vi "RTS Extract Point Array.vi"(8 "Error In":errorcluster, 10 "Chamber Data in":string[][](array[string])=[["System Date", "System Time", "Elapsed Time (sec)", "Elapsed Time (hrs)", "Voltage (V)", "RMS Current (Amps)", "Power (Watts)", "Watt Hours (Wh)", "Voltage Total Harmonic Distortion (%)", "Frequency (Hz)", "Apparent Power (VA)", "Power Factor", "TC 1", "TC 2", "TC 3", "TC 4", "TC 5", "TC 6", "TC 7", "TC 8", "TC 9", "TC 10", "TC 11", "TC 12", "TC 13", "TC 14", "TC 15", "TC 16", "TC 17", "TC 18", "TC 19", "TC 20", "TC 21", "TC 22", "TC 23", "TC 24", "TC 25", "TC 26", "TC 27", "TC 28", "TC 29", "TC 30", "AUX 1", "AUX 2", "CAL CL", "Room Setpoint Temperature", "Room Setpoint Humidity", "Room Temperature (°F)", "Room Humidity (%)", "Door Enable", "Room Setpoint Cool Temperature", "Room Setpoint Dehumidification Temperature", "Supply Temperature (°F)", "Cool Temperature (°F)", "Dehumidification Temperature (°F)", "Glycol Temperature (°F)", "Heat Rate (%)", "Steam Rate (%)", "Cool Rate (%)", "Dehumidification Rate (%)", "Room Status", "Room Dry P", "Room Dry I", "Room Humidity P", "Room Humidity I", "Room Heat P", "Room Heat I", "Room Cool Temperature P", "Room Cool Temperature I", "Room Dehumidification Temperature P", "Room Dehumidification Temperature I", "Voltage Setpoint 1", "60 Hz Power", "50 Hz Power", "120V Range", "240V Range", "Ground Line", "Ground Neutral", "Measure Ground Leakage Current", "Room OK", "S1 Freezer Relay", "S1 Cab Relay", "S1 Slide Relay", "Recording Data", "CVS Location", "Point Location"], ["01/24/2018", "06:36:24.375", "0.000000", "0.000000", "115.046623", "0.030182", "0.135573", "964.507616", "3.000000", "60.021709", "3.472371", "1.000000", "-2.310000", "-1.920000", "-0.910000", "327.670000", "327.670000", "327.670000", "327.670000", "327.670000", "327.670000", "327.670000", "38.020000", "35.660000", "35.030000", "327.670000", "327.670000", "327.670000", "327.670000", "327.670000", "327.670000", "327.670000", "327.670000", "327.670000", "327.670000", "70.360000", "327.670000", "327.670000", "70.300000", "327.670000", "32767.000000", "32767.000000", "0.001000", "0.000000", "1.988000", "70.000000", "35.000000", "70.040000", "38.150000", "1.000000", "55.000000", "48.000000", "66.700000", "55.180000", "48.160000", "0.000000", "36.920000", "0.000000", "30.630000", "8.240000", "0.000000", "200.000000", "15000.000000", "400.000000", "15000.000000", "1000.000000", "2000.000000", "500.000000", "6000.000000", "500.000000", "6000.000000", "115.000000", "1.000000", "0.000000", "1.000000", "0.000000", "0.000000", "1.000000", "0.000000", "1.000000", "0.000000", "0.000000", "0.000000", "FALSE", "", ""], ["System Date", "System Time", "Elapsed Time (sec)", "Elapsed Time (hrs)", "Voltage (V)", "RMS Current (Amps)", "Power (Watts)", "Watt Hours (Wh)", "Voltage Total Harmonic Distortion (%)", "Frequency (Hz)", "Apparent Power (VA)", "Power Factor", "TC 1", "TC 2", "TC 3", "TC 4", "TC 5", "TC 6", "TC 7", "TC 8", "TC 9", "TC 10", "TC 11", "TC 12", "TC 13", "TC 14", "TC 15", "TC 16", "TC 17", "TC 18", "TC 19", "TC 20", "TC 21", "TC 22", "TC 23", "TC 24", "TC 25", "TC 26", "TC 27", "TC 28", "TC 29", "TC 30", "AUX 1", "AUX 2", "CAL CL", "Room Setpoint Temperature", "Room Setpoint Humidity", "Room Temperature (°F)", "Room Humidity (%)", "Door Enable", "Room Setpoint Cool Temperature", "Room Setpoint Dehumidification Temperature", "Supply Temperature (°F)", "Cool Temperature (°F)", "Dehumidification Temperature (°F)", "Glycol Temperature (°F)", "Heat Rate (%)", "Steam Rate (%)", "Cool Rate (%)", "Dehumidification Rate (%)", "Room Status", "Room Dry P", "Room Dry I", "Room Humidity P", "Room Humidity I", "Room Heat P", "Room Heat I", "Room Cool Temperature P", "Room Cool Temperature I", "Room Dehumidification Temperature P", "Room Dehumidification Temperature I", "Voltage Setpoint 2", "60 Hz Power", "50 Hz Power", "120V Range", "240V Range", "Ground Line", "Ground Neutral", "Measure Ground Leakage Current", "Fault", "S2 Freezer Relay", "S2 Cab Relay", "S2 Slide Relay", "Recording Data", "CVS Location", "Point Location"], ["01/24/2018", "06:36:24.375", "0.000000", "0.000000", "114.863785", "0.030740", "0.139474", "26203.680290", "3.500000", "60.021633", "3.530865", "1.000000", "10.000000", "8.600000", "8.210000", "327.670000", "327.670000", "327.670000", "327.670000", "327.670000", "327.670000", "327.670000", "41.900000", "42.090000", "43.130000", "327.670000", "327.670000", "327.670000", "327.670000", "327.670000", "327.670000", "327.670000", "327.670000", "327.670000", "327.670000", "69.920000", "327.670000", "327.670000", "70.410000", "327.670000", "32767.000000", "32767.000000", "0.001000", "0.001000", "1.991000", "70.000000", "35.000000", "70.040000", "38.150000", "1.000000", "55.000000", "48.000000", "66.700000", "55.180000", "48.160000", "0.000000", "36.920000", "0.000000", "30.630000", "8.240000", "0.000000", "200.000000", "15000.000000", "400.000000", "15000.000000", "1000.000000", "2000.000000", "500.000000", "6000.000000", "500.000000", "6000.000000", "115.000000", "1.000000", "0.000000", "1.000000", "0.000000", "0.000000", "1.000000", "0.000000", "0.000000", "0.000000", "0.000000", "0.000000", "FALSE", "", ""], ["System Date", "System Time", "Elapsed Time (sec)", "Elapsed Time (hrs)", "Voltage (V)", "RMS Current (Amps)", "Power (Watts)", "Watt Hours (Wh)", "Voltage Total Harmonic Distortion (%)", "Frequency (Hz)", "Apparent Power (VA)", "Power Factor", "TC 1", "TC 2", "TC 3", "TC 4", "TC 5", "TC 6", "TC 7", "TC 8", "TC 9", "TC 10", "TC 11", "TC 12", "TC 13", "TC 14", "TC 15", "TC 16", "TC 17", "TC 18", "TC 19", "TC 20", "TC 21", "TC 22", "TC 23", "TC 24", "TC 25", "TC 26", "TC 27", "TC 28", "TC 29", "TC 30", "AUX 1", "AUX 2", "CAL CL", "Room Setpoint Temperature", "Room Setpoint Humidity", "Room Temperature (°F)", "Room Humidity (%)", "Door Enable", "Room Setpoint Cool Temperature", "Room Setpoint Dehumidification Temperature", "Supply Temperature (°F)", "Cool Temperature (°F)", "Dehumidification Temperature (°F)", "Glycol Temperature (°F)", "Heat Rate (%)", "Steam Rate (%)", "Cool Rate (%)", "Dehumidification Rate (%)", "Room Status", "Room Dry P", "Room Dry I", "Room Humidity P", "Room Humidity I", "Room Heat P", "Room Heat I", "Room Cool Temperature P", "Room Cool Temperature I", "Room Dehumidification Temperature P", "Room Dehumidification Temperature I", "Voltage Setpoint 3", "60 Hz Power", "50 Hz Power", "120V Range", "240V Range", "Ground Line", "Ground Neutral", "Measure Ground Leakage Current", "Room Heat", "S3 Freezer Relay", "S3 Cab Relay", "S3 Slide Relay", "Recording Data", "CVS Location", "Point Location"], ["01/24/2018", "06:36:24.376", "0.000000", "0.000000", "114.844543", "0.030078", "0.135316", "27955.201782", "3.100000", "60.022556", "3.456682", "1.000000", "0.690000", "0.850000", "2.060000", "327.670000", "327.670000", "327.670000", "327.670000", "327.670000", "327.670000", "327.670000", "37.750000", "38.160000", "38.080000", "327.670000", "327.670000", "327.670000", "327.670000", "327.670000", "327.670000", "327.670000", "327.670000", "327.670000", "327.670000", "70.410000", "327.670000", "327.670000", "70.770000", "327.670000", "32767.000000", "32767.000000", "0.001000", "0.001000", "1.963000", "70.000000", "35.000000", "70.040000", "38.150000", "1.000000", "55.000000", "48.000000", "66.700000", "55.180000", "48.160000", "0.000000", "36.920000", "0.000000", "30.630000", "8.240000", "0.000000", "200.000000", "15000.000000", "400.000000", "15000.000000", "1000.000000", "2000.000000", "500.000000", "6000.000000", "500.000000", "6000.000000", "115.000000", "1.000000", "0.000000", "1.000000", "0.000000", "0.000000", "1.000000", "0.000000", "1.000000", "0.000000", "0.000000", "0.000000", "FALSE", "", ""], ["System Date", "System Time", "Elapsed Time (sec)", "Elapsed Time (hrs)", "Voltage (V)", "RMS Current (Amps)", "Power (Watts)", "Watt Hours (Wh)", "Voltage Total Harmonic Distortion (%)", "Frequency (Hz)", "Apparent Power (VA)", "Power Factor", "TC 1", "TC 2", "TC 3", "TC 4", "TC 5", "TC 6", "TC 7", "TC 8", "TC 9", "TC 10", "TC 11", "TC 12", "TC 13", "TC 14", "TC 15", "TC 16", "TC 17", "TC 18", "TC 19", "TC 20", "TC 21", "TC 22", "TC 23", "TC 24", "TC 25", "TC 26", "TC 27", "TC 28", "TC 29", "TC 30", "AUX 1", "AUX 2", "CAL CL", "Room Setpoint Temperature", "Room Setpoint Humidity", "Room Temperature (°F)", "Room Humidity (%)", "Door Enable", "Room Setpoint Cool Temperature", "Room Setpoint Dehumidification Temperature", "Supply Temperature (°F)", "Cool Temperature (°F)", "Dehumidification Temperature (°F)", "Glycol Temperature (°F)", "Heat Rate (%)", "Steam Rate (%)", "Cool Rate (%)", "Dehumidification Rate (%)", "Room Status", "Room Dry P", "Room Dry I", "Room Humidity P", "Room Humidity I", "Room Heat P", "Room Heat I", "Room Cool Temperature P", "Room Cool Temperature I", "Room Dehumidification Temperature P", "Room Dehumidification Temperature I", "Voltage Setpoint 4", "60 Hz Power", "50 Hz Power", "120V Range", "240V Range", "Ground Line", "Ground Neutral", "Measure Ground Leakage Current", "Room Blower", "S4 Freezer Relay", "S4 Cab Relay", "S4 Slide Relay", "Recording Data", "CVS Location", "Point Location"], ["01/24/2018", "06:36:24.376", "0.000000", "0.000000", "115.200577", "0.030417", "0.136655", "26339.492026", "3.200000", "60.021862", "3.504017", "1.000000", "1.700000", "3.490000", "4.180000", "327.670000", "327.670000", "327.670000", "327.670000", "327.670000", "327.670000", "327.670000", "38.630000", "39.700000", "39.970000", "327.670000", "327.670000", "327.670000", "327.670000", "327.670000", "327.670000", "327.670000", "327.670000", "327.670000", "327.670000", "70.410000", "327.670000", "327.670000", "70.880000", "327.670000", "32767.000000", "32767.000000", "0.001000", "0.000000", "2.005000", "70.000000", "35.000000", "70.040000", "38.150000", "1.000000", "55.000000", "48.000000", "66.700000", "55.180000", "48.160000", "0.000000", "36.920000", "0.000000", "30.630000", "8.240000", "0.000000", "200.000000", "15000.000000", "400.000000", "15000.000000", "1000.000000", "2000.000000", "500.000000", "6000.000000", "500.000000", "6000.000000", "115.000000", "1.000000", "0.000000", "1.000000", "0.000000", "0.000000", "1.000000", "0.000000", "1.000000", "0.000000", "0.000000", "0.000000", "FALSE", "", ""], ["System Date", "System Time", "Elapsed Time (sec)", "Elapsed Time (hrs)", "Voltage (V)", "RMS Current (Amps)", "Power (Watts)", "Watt Hours (Wh)", "Voltage Total Harmonic Distortion (%)", "Frequency (Hz)", "Apparent Power (VA)", "Power Factor", "TC 1", "TC 2", "TC 3", "TC 4", "TC 5", "TC 6", "TC 7", "TC 8", "TC 9", "TC 10", "TC 11", "TC 12", "TC 13", "TC 14", "TC 15", "TC 16", "TC 17", "TC 18", "TC 19", "TC 20", "TC 21", "TC 22", "TC 23", "TC 24", "TC 25", "TC 26", "TC 27", "TC 28", "TC 29", "TC 30", "AUX 1", "AUX 2", "CAL CL", "Room Setpoint Temperature", "Room Setpoint Humidity", "Room Temperature (°F)", "Room Humidity (%)", "Door Enable", "Room Setpoint Cool Temperature", "Room Setpoint Dehumidification Temperature", "Supply Temperature (°F)", "Cool Temperature (°F)", "Dehumidification Temperature (°F)", "Glycol Temperature (°F)", "Heat Rate (%)", "Steam Rate (%)", "Cool Rate (%)", "Dehumidification Rate (%)", "Room Status", "Room Dry P", "Room Dry I", "Room Humidity P", "Room Humidity I", "Room Heat P", "Room Heat I", "Room Cool Temperature P", "Room Cool Temperature I", "Room Dehumidification Temperature P", "Room Dehumidification Temperature I", "Voltage Setpoint 5", "60 Hz Power", "50 Hz Power", "120V Range", "240V Range", "Ground Line", "Ground Neutral", "Measure Ground Leakage Current", "Spare", "S5 Freezer Relay", "S5 Cab Relay", "S5 Slide Relay", "Recording Data", "CVS Location", "Point Location"], ["01/24/2018", "06:36:24.376", "0.000000", "0.000000", "115.123596", "0.000000", "0.000000", "0.000000", "3.300000", "60.022747", "0.000000", "1.000000", "327.670000", "327.670000", "70.410000", "327.670000", "327.670000", "327.670000", "327.670000", "327.670000", "327.670000", "327.670000", "70.630000", "70.360000", "70.360000", "327.670000", "327.670000", "327.670000", "327.670000", "327.670000", "327.670000", "327.670000", "327.670000", "327.670000", "327.670000", "69.950000", "327.670000", "327.670000", "327.670000", "327.670000", "32767.000000", "32767.000000", "0.001000", "0.001000", "1.999000", "70.000000", "35.000000", "70.040000", "38.150000", "1.000000", "55.000000", "48.000000", "66.700000", "55.180000", "48.160000", "0.000000", "36.920000", "0.000000", "30.630000", "8.240000", "0.000000", "200.000000", "15000.000000", "400.000000", "15000.000000", "1000.000000", "2000.000000", "500.000000", "6000.000000", "500.000000", "6000.000000", "115.000000", "1.000000", "0.000000", "1.000000", "0.000000", "0.000000", "1.000000", "0.000000", "0.000000", "0.000000", "0.000000", "0.000000", "FALSE", "", ""], ["System Date", "System Time", "Elapsed Time (sec)", "Elapsed Time (hrs)", "Voltage (V)", "RMS Current (Amps)", "Power (Watts)", "Watt Hours (Wh)", "Voltage Total Harmonic Distortion (%)", "Frequency (Hz)", "Apparent Power (VA)", "Power Factor", "TC 1", "TC 2", "TC 3", "TC 4", "TC 5", "TC 6", "TC 7", "TC 8", "TC 9", "TC 10", "TC 11", "TC 12", "TC 13", "TC 14", "TC 15", "TC 16", "TC 17", "TC 18", "TC 19", "TC 20", "TC 21", "TC 22", "TC 23", "TC 24", "TC 25", "TC 26", "TC 27", "TC 28", "TC 29", "TC 30", "AUX 1", "AUX 2", "CAL CL", "Room Setpoint Temperature", "Room Setpoint Humidity", "Room Temperature (°F)", "Room Humidity (%)", "Door Enable", "Room Setpoint Cool Temperature", "Room Setpoint Dehumidification Temperature", "Supply Temperature (°F)", "Cool Temperature (°F)", "Dehumidification Temperature (°F)", "Glycol Temperature (°F)", "Heat Rate (%)", "Steam Rate (%)", "Cool Rate (%)", "Dehumidification Rate (%)", "Room Status", "Room Dry P", "Room Dry I", "Room Humidity P", "Room Humidity I", "Room Heat P", "Room Heat I", "Room Cool Temperature P", "Room Cool Temperature I", "Room Dehumidification Temperature P", "Room Dehumidification Temperature I", "Voltage Setpoint 6", "60 Hz Power", "50 Hz Power", "120V Range", "240V Range", "Ground Line", "Ground Neutral", "Measure Ground Leakage Current", "Room Pump", "S6 Freezer Relay", "S6 Cab Relay", "S6 Slide Relay", "Recording Data", "CVS Location", "Point Location"], ["01/24/2018", "06:36:24.376", "0.000000", "0.000000", "114.825302", "0.000000", "0.000000", "0.000000", "3.400000", "60.022854", "0.000000", "1.000000", "327.670000", "327.670000", "327.670000", "327.670000", "327.670000", "327.670000", "327.670000", "327.670000", "327.670000", "327.670000", "327.670000", "327.670000", "327.670000", "327.670000", "327.670000", "327.670000", "327.670000", "327.670000", "327.670000", "327.670000", "327.670000", "327.670000", "327.670000", "327.670000", "327.670000", "327.670000", "327.670000", "327.670000", "32767.000000", "32767.000000", "0.001000", "0.001000", "1.995000", "70.000000", "35.000000", "70.040000", "38.150000", "1.000000", "55.000000", "48.000000", "66.700000", "55.180000", "48.160000", "0.000000", "36.920000", "0.000000", "30.630000", "8.240000", "0.000000", "200.000000", "15000.000000", "400.000000", "15000.000000", "1000.000000", "2000.000000", "500.000000", "6000.000000", "500.000000", "6000.000000", "115.000000", "1.000000", "0.000000", "1.000000", "0.000000", "0.000000", "1.000000", "0.000000", "1.000000", "0.000000", "0.000000", "0.000000", "FALSE", "", ""], ["System Date", "System Time", "Elapsed Time (sec)", "Elapsed Time (hrs)", "Voltage (V)", "RMS Current (Amps)", "Power (Watts)", "Watt Hours (Wh)", "Voltage Total Harmonic Distortion (%)", "Frequency (Hz)", "Apparent Power (VA)", "Power Factor", "TC 1", "TC 2", "TC 3", "TC 4", "TC 5", "TC 6", "TC 7", "TC 8", "TC 9", "TC 10", "TC 11", "TC 12", "TC 13", "TC 14", "TC 15", "TC 16", "TC 17", "TC 18", "TC 19", "TC 20", "TC 21", "TC 22", "TC 23", "TC 24", "TC 25", "TC 26", "TC 27", "TC 28", "TC 29", "TC 30", "AUX 1", "AUX 2", "CAL CL", "Room Setpoint Temperature", "Room Setpoint Humidity", "Room Temperature (°F)", "Room Humidity (%)", "Door Enable", "Room Setpoint Cool Temperature", "Room Setpoint Dehumidification Temperature", "Supply Temperature (°F)", "Cool Temperature (°F)", "Dehumidification Temperature (°F)", "Glycol Temperature (°F)", "Heat Rate (%)", "Steam Rate (%)", "Cool Rate (%)", "Dehumidification Rate (%)", "Room Status", "Room Dry P", "Room Dry I", "Room Humidity P", "Room Humidity I", "Room Heat P", "Room Heat I", "Room Cool Temperature P", "Room Cool Temperature I", "Room Dehumidification Temperature P", "Room Dehumidification Temperature I", "Voltage Setpoint 7", "60 Hz Power", "50 Hz Power", "120V Range", "240V Range", "Ground Line", "Ground Neutral", "Measure Ground Leakage Current", "Spare", "S7 Freezer Relay", "S7 Cab Relay", "S7 Slide Relay", "Recording Data", "CVS Location", "Point Location"], ["01/24/2018", "06:36:24.376", "0.000000", "0.000000", "114.796432", "0.000000", "0.000000", "0.000000", "3.500000", "60.023220", "0.000000", "1.000000", "70.630000", "70.630000", "70.630000", "327.670000", "327.670000", "327.670000", "327.670000", "327.670000", "327.670000", "327.670000", "327.670000", "70.300000", "70.300000", "327.670000", "327.670000", "327.670000", "327.670000", "327.670000", "327.670000", "327.670000", "327.670000", "327.670000", "327.670000", "327.670000", "327.670000", "327.670000", "327.670000", "327.670000", "32767.000000", "32767.000000", "0.000000", "0.000000", "2.003000", "70.000000", "35.000000", "70.040000", "38.150000", "1.000000", "55.000000", "48.000000", "66.700000", "55.180000", "48.160000", "0.000000", "36.920000", "0.000000", "30.630000", "8.240000", "0.000000", "200.000000", "15000.000000", "400.000000", "15000.000000", "1000.000000", "2000.000000", "500.000000", "6000.000000", "500.000000", "6000.000000", "115.000000", "1.000000", "0.000000", "1.000000", "0.000000", "0.000000", "1.000000", "0.000000", "0.000000", "0.000000", "0.000000", "0.000000", "FALSE", "", ""], ["System Date", "System Time", "Elapsed Time (sec)", "Elapsed Time (hrs)", "Voltage (V)", "RMS Current (Amps)", "Power (Watts)", "Watt Hours (Wh)", "Voltage Total Harmonic Distortion (%)", "Frequency (Hz)", "Apparent Power (VA)", "Power Factor", "TC 1", "TC 2", "TC 3", "TC 4", "TC 5", "TC 6", "TC 7", "TC 8", "TC 9", "TC 10", "TC 11", "TC 12", "TC 13", "TC 14", "TC 15", "TC 16", "TC 17", "TC 18", "TC 19", "TC 20", "TC 21", "TC 22", "TC 23", "TC 24", "TC 25", "TC 26", "TC 27", "TC 28", "TC 29", "TC 30", "AUX 1", "AUX 2", "CAL CL", "Room Setpoint Temperature", "Room Setpoint Humidity", "Room Temperature (°F)", "Room Humidity (%)", "Door Enable", "Room Setpoint Cool Temperature", "Room Setpoint Dehumidification Temperature", "Supply Temperature (°F)", "Cool Temperature (°F)", "Dehumidification Temperature (°F)", "Glycol Temperature (°F)", "Heat Rate (%)", "Steam Rate (%)", "Cool Rate (%)", "Dehumidification Rate (%)", "Room Status", "Room Dry P", "Room Dry I", "Room Humidity P", "Room Humidity I", "Room Heat P", "Room Heat I", "Room Cool Temperature P", "Room Cool Temperature I", "Room Dehumidification Temperature P", "Room Dehumidification Temperature I", "Voltage Setpoint 8", "60 Hz Power", "50 Hz Power", "120V Range", "240V Range", "Ground Line", "Ground Neutral", "Measure Ground Leakage Current", "Spare", "S8 Freezer Relay", "S8 Cab Relay", "S8 Slide Relay", "Recording Data", "CVS Location", "Point Location"], ["01/24/2018", "06:36:24.377", "0.000000", "0.000000", "115.306419", "0.000000", "0.000000", "0.000000", "3.500000", "60.021893", "0.000000", "1.000000", "70.630000", "70.440000", "70.490000", "327.670000", "327.670000", "327.670000", "327.670000", "327.670000", "327.670000", "327.670000", "70.630000", "70.410000", "70.300000", "327.670000", "327.670000", "327.670000", "327.670000", "327.670000", "327.670000", "327.670000", "327.670000", "327.670000", "327.670000", "327.670000", "327.670000", "327.670000", "327.670000", "327.670000", "32767.000000", "32767.000000", "0.000000", "0.000000", "1.955000", "70.000000", "35.000000", "70.040000", "38.150000", "1.000000", "55.000000", "48.000000", "66.700000", "55.180000", "48.160000", "0.000000", "36.920000", "0.000000", "30.630000", "8.240000", "0.000000", "200.000000", "15000.000000", "400.000000", "15000.000000", "1000.000000", "2000.000000", "500.000000", "6000.000000", "500.000000", "6000.000000", "115.000000", "1.000000", "0.000000", "1.000000", "0.000000", "0.000000", "1.000000", "0.000000", "0.000000", "0.000000", "0.000000", "0.000000", "FALSE", "", ""]], 11 "Tree Selection in":T1) -> (0 "Error Out":errorcluster, 3 "Chamber Data out":string[][](array[string]))   [LabVIEW 2020]
uses:
  Type Definitions/RTS Room Selector.ctl
  <vilib>/Utility/error.llb/whitespace.ctl
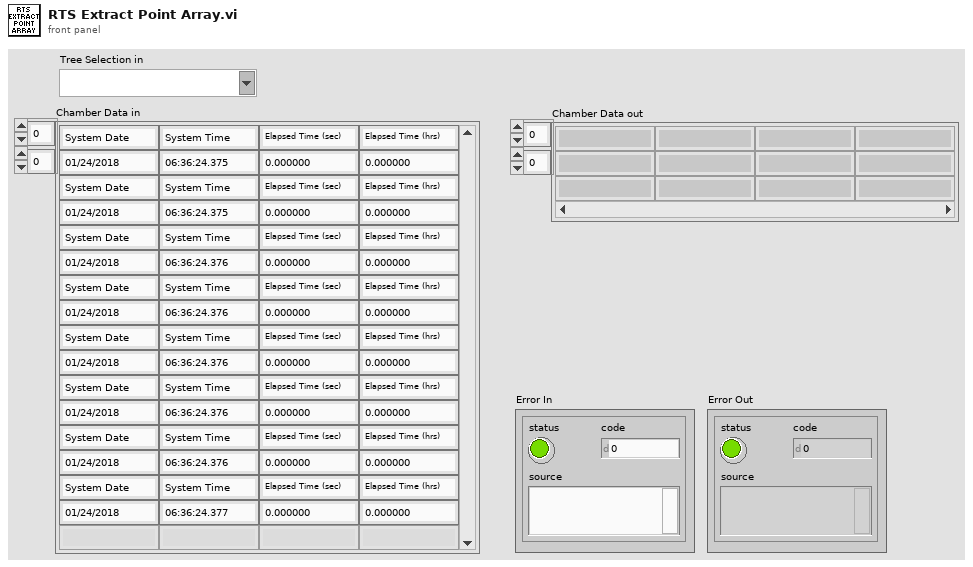
[diagram p1: front panel]
types:
  T1 = typedef "RTS Room Selector.ctl" = string
  T2 = typedef "whitespace.ctl" = u16
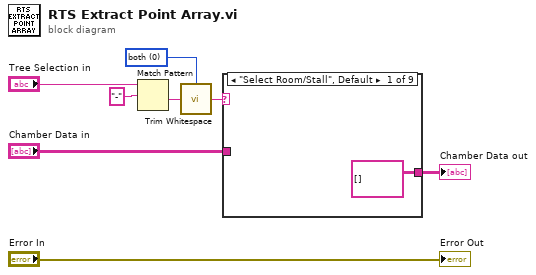
[diagram p0: block diagram]
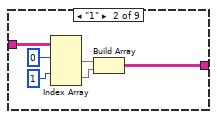
[diagram p2: hidden frame]
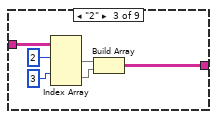
[diagram p3: hidden frame]
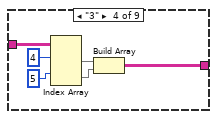
[diagram p4: hidden frame]
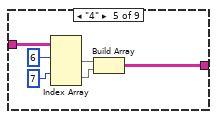
[diagram p5: hidden frame]
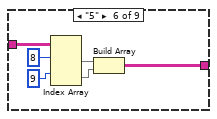
[diagram p6: hidden frame]
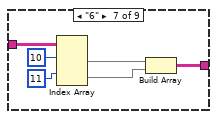
[diagram p7: hidden frame]
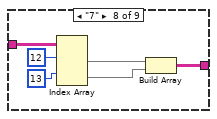
[diagram p8: hidden frame]
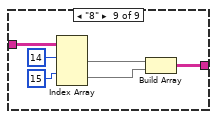
[diagram p9: hidden frame]
diagram:
  w6 = T2 0 items=["both", "start of string", "end of string"] ("location (both)")
  n1 = Match Pattern(string="Tree Selection in", regular expression="-") -> (after substring=w5:T1)  [unwired: 1 in, 3 out]
  n2 = call <vilib>:"Trim Whitespace.vi"("string"=w5, "location (both)"=w6) -> ("trimmed string"=w7:string)
  n3 = case shown="\"Select Room/Stall\", Default" w7 {
    tunnel: "Chamber Data in" -> [_ w11 w17 w23 w28 w35 w41 w47 w53]
    tunnel: [string[][] [] ("Chamber Data") w10 w16 w22 w29 w34 w40 w46 w52] -> w8
    frame "Select Room/Stall", Default {
    }
    frame "1" {
      n4 = Index Array(array=w11, index (row) #1=0 ("index (row)"), index (row) #2=1 ("index (row)")) -> (element #1=w13:string[], element #2=w12:string[])  [unwired: 2 in]
      n5 = Build Array(w13, w12) -> (w10:string[][])
    }
    frame "2" {
      n6 = Index Array(array=w17, index (row) #1=2 ("index (row)"), index (row) #2=3 ("index (row)")) -> (element #1=w19:string[], element #2=w18:string[])  [unwired: 2 in]
      n7 = Build Array(w19, w18) -> (w16:string[][])
    }
    frame "3" {
      n8 = Index Array(array=w23, index (row) #1=4 ("index (row)"), index (row) #2=5 ("index (row)")) -> (element #1=w25:string[], element #2=w24:string[])  [unwired: 2 in]
      n9 = Build Array(w25, w24) -> (w22:string[][])
    }
    frame "4" {
      n10 = Index Array(array=w28, index (row) #1=6 ("index (row)"), index (row) #2=7 ("index (row)")) -> (element #1=w31:string[], element #2=w30:string[])  [unwired: 2 in]
      n11 = Build Array(w31, w30) -> (w29:string[][])
    }
    frame "5" {
      n12 = Index Array(array=w35, index (row) #1=8 ("index (row)"), index (row) #2=9 ("index (row)")) -> (element #1=w37:string[], element #2=w36:string[])  [unwired: 2 in]
      n13 = Build Array(w37, w36) -> (w34:string[][])
    }
    frame "6" {
      n14 = Index Array(array=w41, index (row) #1=10 ("index (row)"), index (row) #2=11 ("index (row)")) -> (element #1=w43:string[], element #2=w42:string[])  [unwired: 2 in]
      n15 = Build Array(w43, w42) -> (w40:string[][])
    }
    frame "7" {
      n16 = Index Array(array=w47, index (row) #1=12 ("index (row)"), index (row) #2=13 ("index (row)")) -> (element #1=w49:string[], element #2=w48:string[])  [unwired: 2 in]
      n17 = Build Array(w49, w48) -> (w46:string[][])
    }
    frame "8" {
      n18 = Index Array(array=w53, index (row) #1=14 ("index (row)"), index (row) #2=15 ("index (row)")) -> (element #1=w55:string[], element #2=w54:string[])  [unwired: 2 in]
      n19 = Build Array(w55, w54) -> (w52:string[][])
    }
  }
  "Chamber Data out" <- w8
  "Error Out" <- "Error In"
